vi "Intan_1dstream_to_2d_samps_128ch.vi"(0 "1-D  data in":u16[](array[numeric]), 5 "Nchans":i32=64, 9 "N data scans to read":i32=1, 11 "bytes per scan":i32=148) -> (3 "fragmented frame read":bool, 4 "2d ADCdata_array out_ampA_and_B":u16[][](array[numeric]), 6 "timestamp_array":i32[](array[numeric]), 8 "Nscans read":i32, 10 "aux_cmd_array A_and_B":i16[][](array[numeric]), 12 "ADXL analog data out":u16[][](array[numeric]), 14 "Nscans underflow":bool, 15 "SyncBytes Out":i32[](array[numeric]))   [LabVIEW 2017]
doc: "Reformats a 1d array of U16 Intan data (written by Teensy to serial port) into a 2-D array of data.\nThis takes Nscans worth of data, each with 36 words (= 72 bytes) worth of data, and reformats into 3 arrays:\n1. 'IN' = [73, 78] ascii values from auxiliary commands (this can be checked to verify data link)\n2. 32 bit timestamp (microseconds)\n3. Nchans (=32 for now) U16s for ADC data, with data formatted as Nchans x Nsamps\n\nRead error indicators suggest possible mis-read/mis-handling of data"
panel:
  # "Data format for 64 chan + adxl:\n4 bytes aux_cmd_A\n4 bytes aux_cmd_B\n4 bytes timestamp\n64 bytes ADC amp A\n64 bytes ADC amp B\n6 bytes ADXL (x,y,z)\n2 bytes sync bits\n------------------\n148 bytes total"
  # "2-D data output"
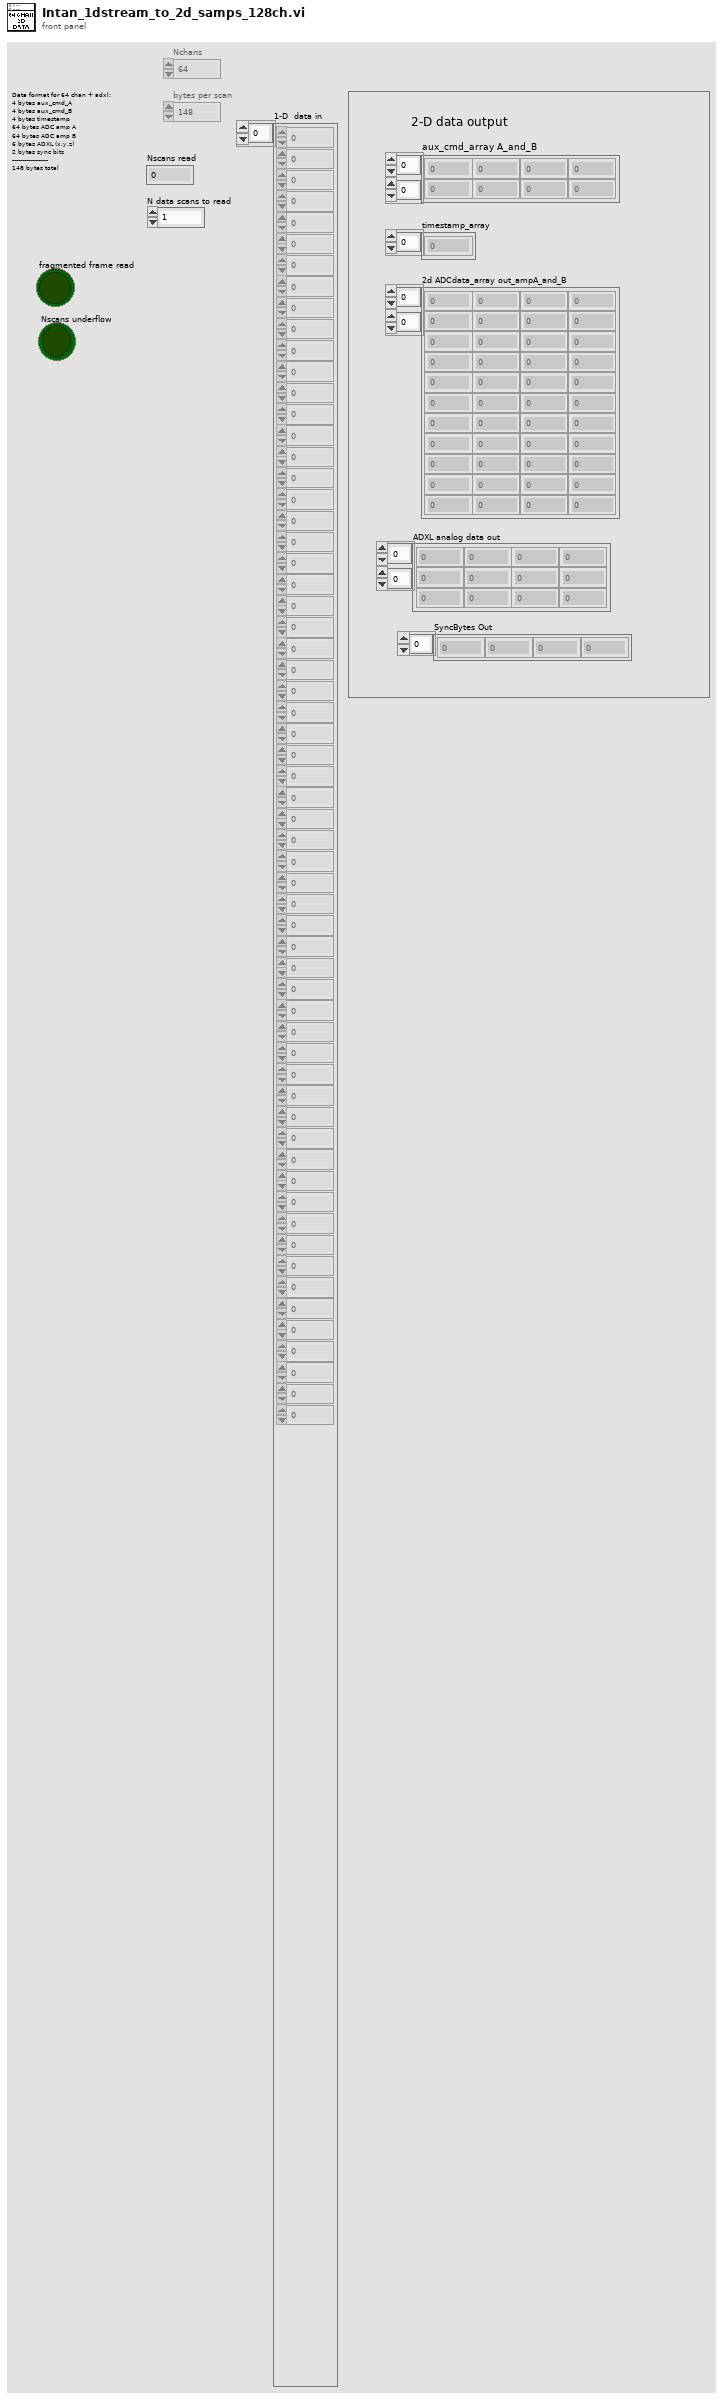
[diagram p1: front panel]
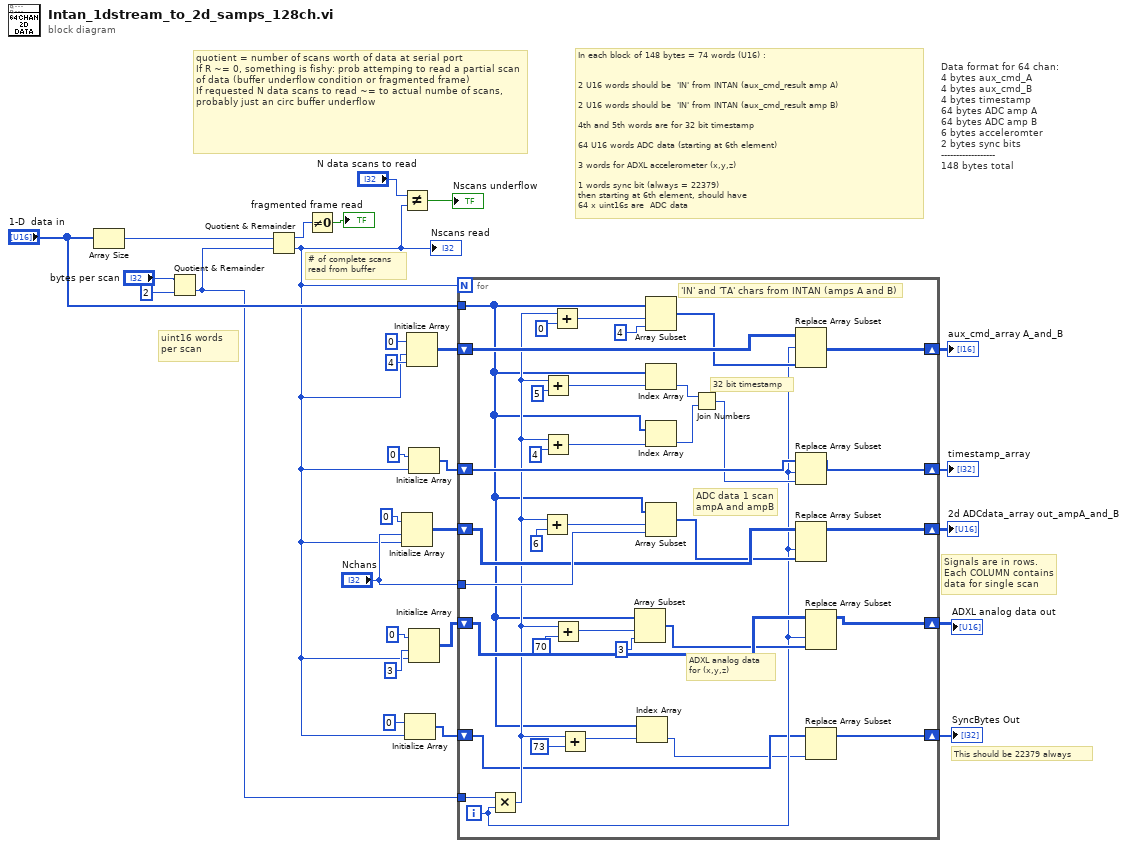
[diagram p0: block diagram]
diagram:
  # "This should be 22379 always"
  # "Data format for 64 chan:\n4 bytes aux_cmd_A\n4 bytes aux_cmd_B\n4 bytes timestamp\n64 bytes ADC amp A\n64 bytes ADC amp B\n6 bytes acceleromter\n2 bytes sync bits\n------------------\n148 bytes total"
  # "# of complete scans\nread from buffer"
  # "Signals are in rows.\nEach COLUMN contains\ndata for single scan"
  # "In each block of 148 bytes = 74 words (U16) :\n\n\n2 U16 words should be  'IN' from INTAN (aux_cmd_result amp A)\n\n2 U16 words should be  'IN' from INTAN (aux_cmd_result amp B)\n\n4th and 5th words are for 32 bit timestamp\n\n64 U16 words ADC data (starting at 6th element)\n\n3 words for ADXL accelerometer (x,y,z)\n\n1 words sync bit (always = 22379)\nthen starting at 6th element, should have\n64 x uint16s are  ADC data"
  # "quotient = number of scans worth of data at serial port \nIf R ~= 0, something is fishy: prob attemping to read a partial scan of data (buffer underflow condition or fragmented frame)\nIf requested N data scans to read ~= to actual numbe of scans, probably just an circ buffer underflow"
  # "uint16 words per scan"
  n1 = Array Size(array="1-D  data in") -> (size(s)=w27:i32)
  n2 = Quotient & Remainder(x="bytes per scan", y=2) -> (floor(x/y)=w22:i32)  [unwired: 1 out]
  n3 = Quotient & Remainder(x=w27, y=w22) -> (x-y*floor(x/y)=w26:i32, floor(x/y)=w1:i32)
  "Nscans read" <- w1
  n4 = Not Equal To 0?(x=w26) -> (x != 0?=→"fragmented frame read":bool)
  n5 = Not Equal?(x="N data scans to read", y=w1) -> (x != y?=→"Nscans underflow":bool)
  n6 = Initialize Array(u16 0 ("element"), "Nchans", w1) -> (w15:u16[][])
  n7 = Initialize Array(0 ("element"), w1) -> (w4:i32[])
  n8 = Initialize Array(0 ("element"), w1, 4 ("dimension size")) -> (w17:i32[][])
  n9 = Initialize Array(0 ("element"), w1) -> (w16:i32[])
  n10 = Initialize Array(u16 0 ("element"), 3 ("dimension size"), w1) -> (w6:u16[][])
  n11 = for {
    N: w1 -> [_]
    tunnel: "1-D  data in" -> [w31]
    tunnel: w22 -> [w61]
    tunnel: "Nchans" -> [w52]
    shift-right: [w47] -> w10
    shift-left: w16 -> [w50]
    shift-right: [w49] -> w11
    shift-left: w17 -> [w51]
    shift-right: [w46] -> w9
    shift-left: w15 -> [w48]
    shift-right: [w36] -> w5
    shift-left: w6 -> [w39]
    shift-right: [w33] -> w2
    shift-left: w4 -> [w32]
    i -> [w37]
    # "ADXL analog data\nfor (x,y,z)"
    # "ADC data 1 scan\nampA and ampB"
    # "'IN' and 'TA' chars from INTAN (amps A and B)"
    # "32 bit timestamp"
    n12 = Multiply(x=w61, y=w37) -> (x*y=w35:i32)
    n13 = Add(x=w35, y=6 ("index")) -> (x+y=w53:i32)
    n14 = Add(x=w35, y=5 ("index")) -> (x+y=w55:i32)
    n15 = Add(x=w35, y=4 ("index")) -> (x+y=w54:i32)
    n16 = Add(x=w35, y=0 ("index")) -> (x+y=w56:i32)
    n17 = Add(x=w35, y=70 ("index")) -> (x+y=w40:i32)
    n18 = Add(x=w35, y=73) -> (x+y=w30:i32)
    n19 = Array Subset(array=w31, index=w40, length=3) -> (w38:u16[])
    n20 = Index Array(array=w31, index=w30) -> (element=w29:u16)
    n21 = Array Subset(array=w31, index=w56, length=4) -> (w45:u16[])
    n22 = Index Array(array=w31, index=w55) -> (element=w63:u16)
    n23 = Index Array(array=w31, index=w54) -> (element=w62:u16)
    n24 = Array Subset(array=w31, index=w53, length=w52) -> (w43:u16[])
    n25 = Join Numbers(hi=w63, lo=w62) -> ((hi.lo)=w44:u32)
    n26 = Replace Array Subset(array=w51, new element=w45, index (row)=w37) -> (w49:i32[][])  [unwired: 1 in]
    n27 = Replace Array Subset(array=w50, new element=w44, index=w37) -> (w47:i32[])
    n28 = Replace Array Subset(array=w48, new element=w43, index (col)=w37) -> (w46:u16[][])  [unwired: 1 in]
    n29 = Replace Array Subset(array=w39, new element=w38, index (col)=w37) -> (w36:u16[][])  [unwired: 1 in]
    n30 = Replace Array Subset(array=w32, new element=w29) -> (w33:i32[])  [unwired: 1 in]
  }
  "aux_cmd_array A_and_B" <- w11
  "timestamp_array" <- w10
  "2d ADCdata_array out_ampA_and_B" <- w9
  "ADXL analog data out" <- w5
  "SyncBytes Out" <- w2
